vi "FPGA VeriStand Native DMA Interface.vi"() -> ()   [LabVIEW 2017]
uses:
  <vilib>/Platform/TimedLoop/XDataNode/timing_clust.ctl
  <vilib>/Platform/TimedLoop/XDataNode/nitl_modes.ctl
  <vilib>/Platform/TimedLoop/XDataNode/wakeup.ctl
  <vilib>/rvi/Emulation/niFpgaSctlEmulationGetInTimedLoop.vi
  <vilib>/rvi/Emulation/niFpgaEmulationReportErrorSimple.vi
  <vilib>/rvi/Emulation/niFpgaGetClockAttributes.vi
  <vilib>/rvi/Emulation/niFpgaCriticalErrorInLSC.vi
  <vilib>/rvi/eio/common/nirviEmuTemplateMethod_errors.vi
  <vilib>/rvi/Emulation/niFpgaProcessEmulError.vi
  <vilib>/Platform/TimedLoop/XDataNode/XDataNode.xnode
  <vilib>/eio/EIONode/EIONode.xnode
  <vilib>/eio/EIOMethodNode/EIOMethodNode.xnode
  <vilib>/Platform/TimedLoop/XDataNode/XDNodeRunTimeDep.lvlib
  <vilib>/NI Veristand/FPGA/NI_VS FPGA Support.lvlib
panel:
  in  "Generate IRQ":bool
  in  "Clock Pulse":bool
  in  "Clock Ticked":bool
  in  "Use External Timing":bool
  in  "Write to  RTSI":bool
  in  "Loop Rate (usec)":u32
  in  "Start":bool
  in  "_PWM In 1 timeout":u32=40000
  out "_PWM In 1 High Time":u32
  out "_PWM In 1 Low Time":u32
  in  "_PWM In 0 timeout":u32=40000
  out "_PWM In 0 High Time":u32
  out "_PWM In 0 Low Time":u32
  in  "_Low Pulse 1":u32
  in  "_High Pulse 1":u32
  in  "_Low Pulse 0":u32
  in  "_High Pulse 0":u32
  # "PWM"
  # "Configuration"
  # "Internal Controls"
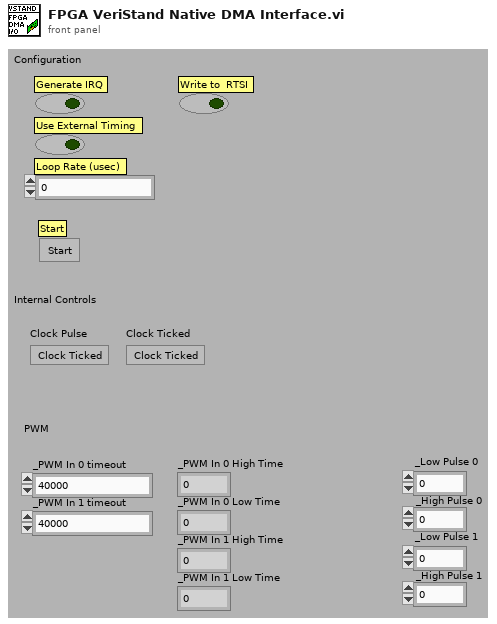
[diagram p1: front panel]
types:
  T1 = typedef "XDNodeRunTimeDep.lvlib/timing_clust.ctl" = cluster{"Expected End [f-1]":u64, "Actual End [f-1]":u64, "Finished Late? [f-1]":bool, "Expected End [i-1]":u64, "Actual End [i-1]":u64, "Finished Late? [i-1]":bool, "Expected Start [i]":u64, "Actual Start [i]":u64, "Expected Start [f]":u64, "Actual Start [f]":u64, "Source Name":string, "Structure Name":string, "Period":i64, "Deadline":i64, "Offset":i64, "Start":i64, "Priority":i32, "Timeout":i32, "Mode":T2, "Wakeup Reason":T3, "Error":errorcluster, "Source Type":string, "Secondary Source Type":string, "Global End Time":u64, "Global Start Time":u64, "Frame Duration":u64, "Iteration Duration":u64, "Assigned CPU":i32, "I/O Scan Engine Mode":u32}
  T2 = typedef "XDNodeRunTimeDep.lvlib/nitl_modes.ctl" = enum32{"No Change", "Process missed periods, maintain original phase", "Discard missed periods, maintain original phase", "Process missed periods, ignore original phase", "Discard missed periods, ignore original phase"}
  T3 = typedef "XDNodeRunTimeDep.lvlib/wakeup.ctl" = enum32{"Normal", "Aborted", "Asynchronous wakeup", "Timing source error", "Timed loop error", "Timeout"}
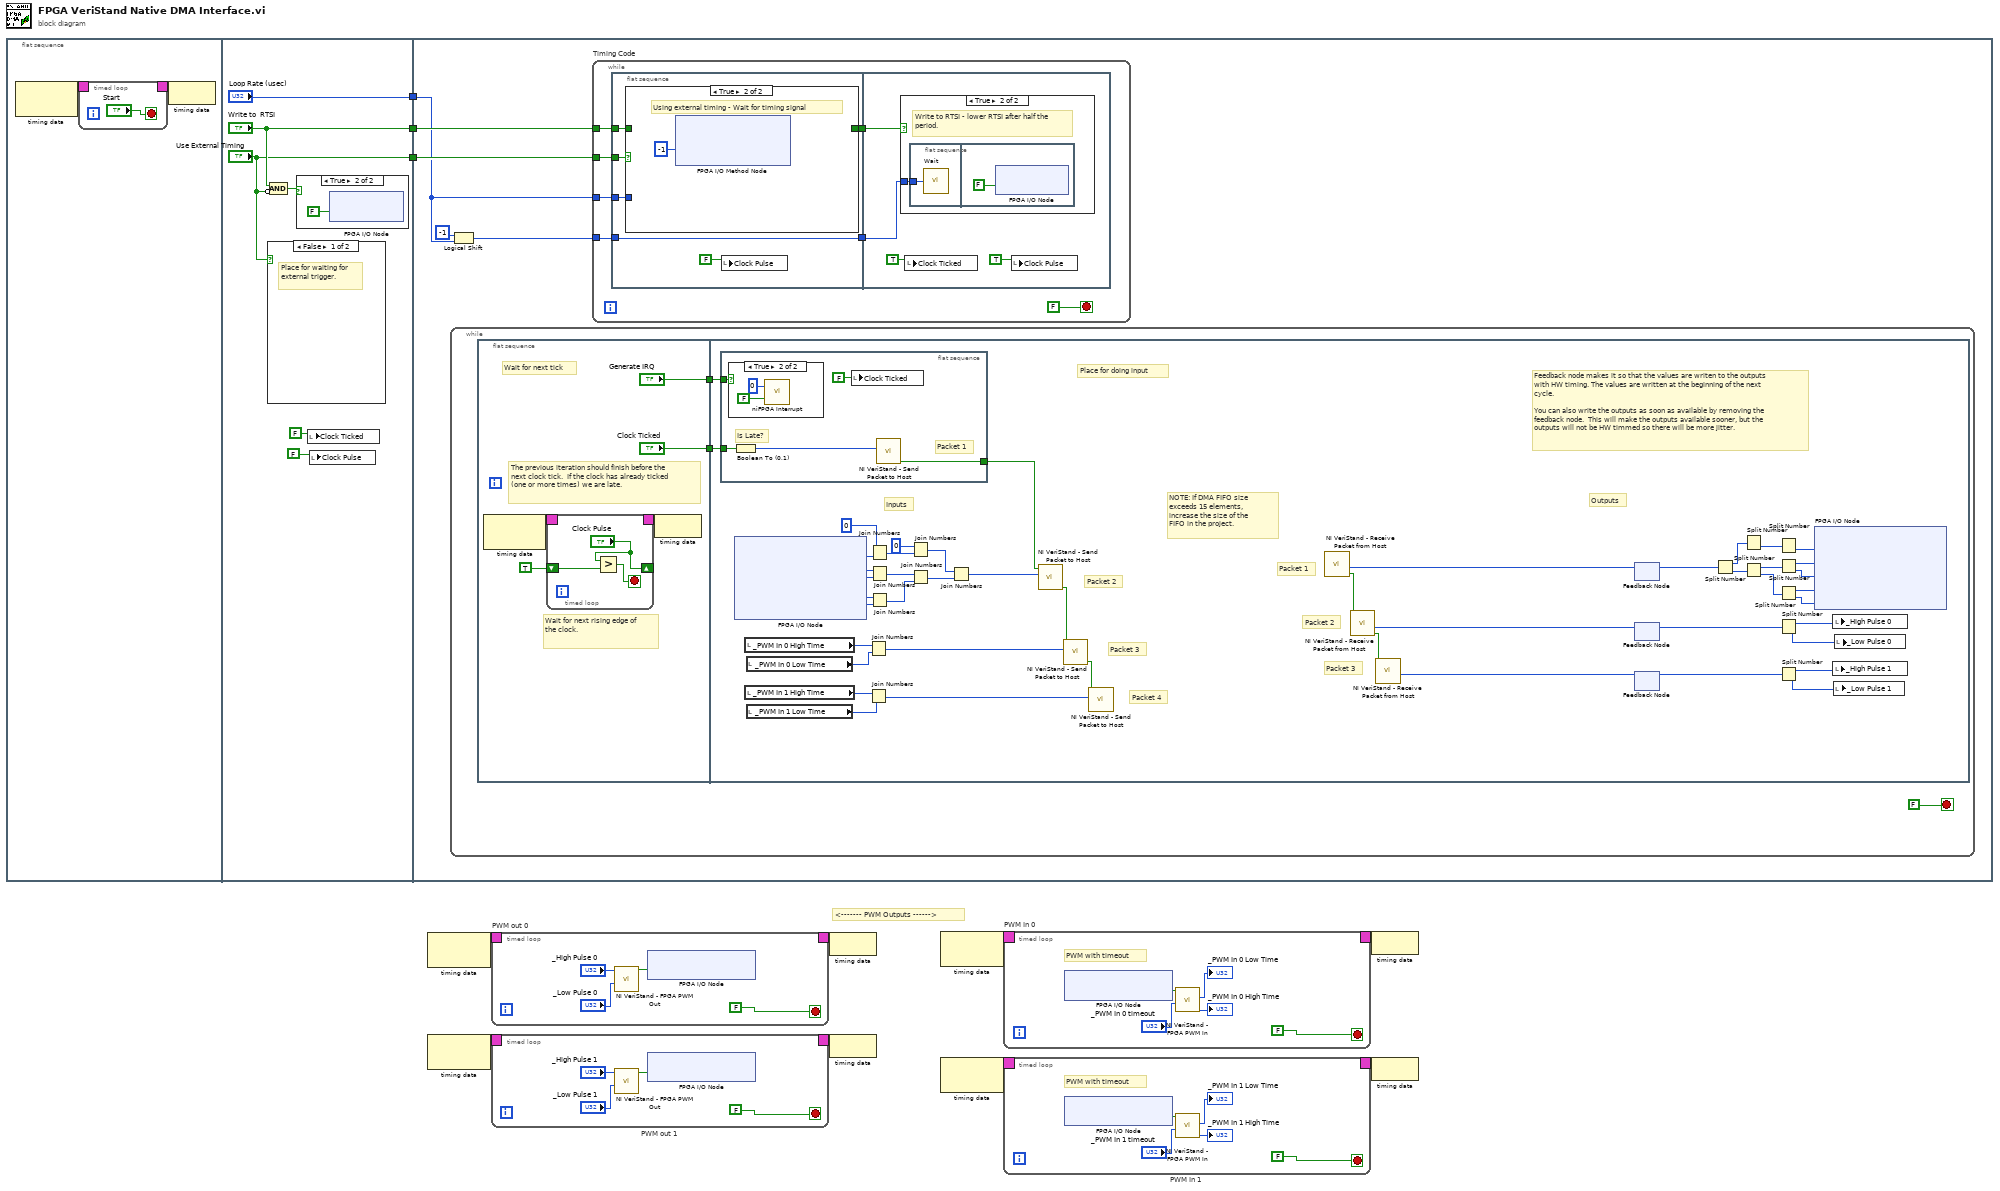
[diagram p0: block diagram]
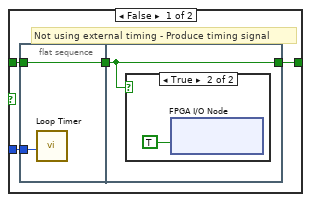
[diagram p4: hidden frame]
diagram:
  # "<------- PWM Outputs ------>"
  n1 = flat-sequence {
    tunnel: ["Use External Timing"] -> w3
    tunnel: ["Write to  RTSI"] -> w2
    tunnel: ["Loop Rate (usec)"] -> w1
    tunnel: w3 -> [w28]
    tunnel: w2 -> [w27]
    tunnel: w1 -> [w26]
    frame #0 {
      n2 = node-c288() -> (w13:T1)  [unwired: 1 out]
      n3 = timed-loop {
        timing: w13 -> [_]
        timing-out: [_] -> w12
        stop <- "Start" stop-if-true
      }
      n4 = node-c288(w12) -> ()
    }
    frame #1 {
      n5 = case shown="False" "Use External Timing" {
        frame False {
          # "Place for waiting for external trigger."
        }
        frame True {
          # "Do not wait on trigger when externally timed."
        }
      }
      n6 = Compound Arithmetic op=AND("Write to  RTSI", invert "Use External Timing") -> (w23:bool)
      n7 = case shown="True" w23 {
        frame False {
        }
        frame True {
          n8 = xnode "FPGA I/O Node"("PXI_Trig0"=FALSE ("TRIG0")) -> ()  [unwired: 1 in, 1 out]
        }
      }
      n9 = local write "Clock Ticked"(FALSE ("Clock Ticked")) -> ()
      n10 = local write "Clock Pulse"(FALSE ("Clock Ticked")) -> ()
    }
    frame #2 {
      n11 = Logical Shift(y=i8 -1, x=w26) -> (x << y=w29:u32)
      n12 = while {
        stop <- FALSE stop-if-true
        n13 = flat-sequence {
          tunnel: ["Generate IRQ"] -> w61
          tunnel: ["Clock Ticked"] -> w60
          tunnel: w61 -> [w120]
          tunnel: w60 -> [w119]
          frame #0 {
            # "The previous iteration should finish before the next clock tick.  If the clock has already ticked (one or more times) we are late."
            # "Wait for next rising edge of the clock."
            # "Wait for next tick"
            n14 = node-c288() -> (w66:T1)  [unwired: 1 out]
            n15 = timed-loop {
              timing: w66 -> [_]
              timing-out: [_] -> w65
              shift-right: ["Clock Pulse"] -> _
              shift-left: TRUE ("Clock Ticked") -> [w70]
              stop <- w69 stop-if-true
              n16 = Greater?(x="Clock Pulse", y=w70) -> (0:w69:bool)
            }
            n17 = node-c288(w65) -> ()
          }
          frame #1 {
            # "Inputs"
            # "Outputs"
            # "Packet 4"
            # "Packet 3"
            # "Packet 2"
            # "Packet 3"
            # "Packet 2"
            # "Packet 1"
            # "NOTE: If DMA FIFO size exceeds 15 elements, increase the size of the FIFO in the project."
            # "Feedback node makes it so that the values are writen to the outputs with HW timing. The values are written at the beginning of the next cycle.  \n\nYou can also write the outputs as soon as available by removing the feedback node.  This will make the outputs available sooner, but the outputs will not be HW timmed so there will be more jitter."
            # "Place for doing input"
            n18 = flat-sequence {
              tunnel: w120 -> [w125]
              tunnel: [w123] -> w75
              tunnel: w119 -> [w121]
              frame #0 {
                # "Packet 1"
                # "Is Late?"
                n19 = case shown="True" w125 {
                  frame False {
                  }
                  frame True {
                    n20 = call <vilib>:"niFPGA Interrupt.vi"("Wait Until Cleared (F)"=FALSE ("Wait Until Cleared"), "IRQ Number (0)"=u8 0 ("IRQ Number")) -> ()  [unwired: 1 in]
                  }
                }
                n21 = Boolean To (0,1)(Boolean=w121) -> (0, 1=w124:i16)
                n22 = local write "Clock Ticked"(FALSE ("Clock Ticked")) -> ()
                n23 = call <vilib>:"NI VeriStand - Send Packet to Host.vi"("Element"=w124) -> ("Next"=w123:bool)  [unwired: 1 in, 9 out]
              }
            }
            n24 = xnode "FPGA I/O Node"() -> ("Connector1/DIOPORT3"=w118:u8, "Connector1/DIOPORT3"=w117:u8, "Connector1/DIOPORT2"=w116:u8, "Connector1/DIOPORT1"=w115:u8, "Connector1/DIOPORT0"=w114:u8)  [unwired: 5 in, 5 out]
            n25 = local read "_PWM In 0 High Time"() -> (w108:u32)
            n26 = local read "_PWM In 1 High Time"() -> (w106:u32)
            n27 = local read "_PWM In 0 Low Time"() -> (w107:u32)
            n28 = local read "_PWM In 1 Low Time"() -> (w105:u32)
            n29 = Join Numbers(hi=w108, lo=w107) -> ((hi.lo)=w87:u64)
            n30 = Join Numbers(hi=w106, lo=w105) -> ((hi.lo)=w86:u64)
            n31 = Join Numbers(hi=u8 0, lo=w118) -> ((hi.lo)=w113:u16)
            n32 = Join Numbers(hi=w117, lo=w116) -> ((hi.lo)=w112:u16)
            n33 = Join Numbers(hi=w115, lo=w114) -> ((hi.lo)=w111:u16)
            n34 = Join Numbers(hi=u16 0, lo=w113) -> ((hi.lo)=w110:u32)
            n35 = Join Numbers(hi=w112, lo=w111) -> ((hi.lo)=w109:u32)
            n36 = Join Numbers(hi=w110, lo=w109) -> ((hi.lo)=w88:u64)
            n37 = call <vilib>:"NI VeriStand - Send Packet to Host.vi"("Element"=w88, "Prev"=w75) -> ("Next"=w77:bool)  [unwired: 1 in, 8 out]
            n38 = call <vilib>:"NI VeriStand - Send Packet to Host.vi"("Element"=w87, "Prev"=w77) -> ("Next"=w76:bool)  [unwired: 1 in, 8 out]
            n39 = call <vilib>:"NI VeriStand - Send Packet to Host.vi"("Element"=w86, "Prev"=w76) -> ()  [unwired: 1 in, 9 out]
            n40 = call <vilib>:"NI VeriStand - Receive Packet from Host.vi"() -> ("Next"=w79:bool, "Element"=w85:u64)  [unwired: 2 in, 8 out]
            n41 = call <vilib>:"NI VeriStand - Receive Packet from Host.vi"("Prev"=w79) -> ("Next"=w78:bool, "Element"=w84:u64)  [unwired: 1 in, 8 out]
            n42 = call <vilib>:"NI VeriStand - Receive Packet from Host.vi"("Prev"=w78) -> ("Element"=w83:u64)  [unwired: 1 in, 9 out]
            n43 = feedback-in #1(w85) -> ()
            n44 = feedback #1() -> (w82:u64)  [unwired: 1 out]
            n45 = feedback-in #2(w84) -> ()
            n46 = feedback #2() -> (w81:u64)  [unwired: 1 out]
            n47 = feedback-in #3(w83) -> ()
            n48 = feedback #3() -> (w80:u64)  [unwired: 1 out]
            n49 = Split Number(x=w82) -> (hi(x)=w99:u32, lo(x)=w98:u32)
            n50 = Split Number(x=w99) -> (lo(x)=w100:u16)  [unwired: 1 out]
            n51 = Split Number(x=w98) -> (hi(x)=w102:u16, lo(x)=w101:u16)
            n52 = Split Number(x=w100) -> (lo(x)=w89:u8)  [unwired: 1 out]
            n53 = Split Number(x=w102) -> (hi(x)=w90:u8, lo(x)=w91:u8)
            n54 = Split Number(x=w101) -> (hi(x)=w92:u8, lo(x)=w93:u8)
            n55 = Split Number(x=w81) -> (hi(x)=w97:u32, lo(x)=w96:u32)
            n56 = Split Number(x=w80) -> (hi(x)=w95:u32, lo(x)=w94:u32)
            n57 = xnode "FPGA I/O Node"("Connector0/DIOPORT0"=w89, "Connector0/DIOPORT1"=w90, "Connector0/DIOPORT0"=w91, "Connector0/DIOPORT1"=w92, "Connector0/DIOPORT0"=w93) -> ()  [unwired: 5 in, 5 out]
            n58 = local write "_High Pulse 0"(w97) -> ()
            n59 = local write "_High Pulse 1"(w95) -> ()
            n60 = local write "_Low Pulse 1"(w94) -> ()
            n61 = local write "_Low Pulse 0"(w96) -> ()
          }
        }
      }
      n62 = while "Timing Code" {
        tunnel: w29 -> [w37]
        tunnel: w26 -> [w36]
        tunnel: w28 -> [w35]
        tunnel: w27 -> [w34]
        stop <- FALSE stop-if-true
        n63 = flat-sequence {
          tunnel: w37 -> [w40]
          tunnel: w36 -> [w43]
          tunnel: w35 -> [w42]
          tunnel: w34 -> [w41]
          tunnel: [w40] -> w32
          tunnel: [w38] -> w31
          tunnel: w32 -> [w56]
          tunnel: w31 -> [w53]
          frame #0 {
            n64 = case shown="True" w42 {
              tunnel: w43 -> [w47 _]
              tunnel: w41 -> [w45 _]
              tunnel: [w44 _] -> w38
              frame False {
                # "Not using external timing - Produce timing signal"
                n65 = flat-sequence {
                  tunnel: [w48] -> w46
                  tunnel: w47 -> [w49]
                  tunnel: w45 -> [w48]
                  tunnel: w46 -> [w50]
                  tunnel: [w50] -> w44
                  frame #0 {
                    n66 = call "Loop Timer"("Count(uSec)"=w49) -> ()  [unwired: 1 out]
                  }
                  frame #1 {
                    n67 = case shown="True" w50 {
                      frame False {
                      }
                      frame True {
                        n68 = xnode "FPGA I/O Node"("PXI_Trig0"=TRUE ("TRIG0")) -> ()  [unwired: 1 in, 1 out]
                      }
                    }
                  }
                }
              }
              frame True {
                # "Using external timing - Wait for timing signal"
                n69 = xnode "FPGA I/O Method Node"("Timeout"=-1) -> ()  [unwired: 1 in, 2 out]
              }
            }
            n70 = local write "Clock Pulse"(FALSE ("Clock Ticked")) -> ()
          }
          frame #1 {
            n71 = case shown="True" w53 {
              tunnel: w56 -> [_ w57]
              frame False {
              }
              frame True {
                # "Write to RTSI - lower RTSI after half the period."
                n72 = flat-sequence {
                  tunnel: w57 -> [w58]
                  frame #0 {
                    n73 = call "Wait"("Count(uSec)"=w58) -> ()  [unwired: 1 out]
                  }
                  frame #1 {
                    n74 = xnode "FPGA I/O Node"("PXI_Trig0"=FALSE ("TRIG0")) -> ()  [unwired: 1 in, 1 out]
                  }
                }
              }
            }
            n75 = local write "Clock Ticked"(TRUE ("Clock Ticked")) -> ()
            n76 = local write "Clock Pulse"(TRUE ("Clock Ticked")) -> ()
          }
        }
      }
    }
  }
  n77 = node-c288() -> (w11:T1)  [unwired: 1 out]
  n78 = node-c288() -> (w9:T1)  [unwired: 1 out]
  n79 = timed-loop "PWM out 0" {
    timing: w11 -> [_]
    timing-out: [_] -> w10
    stop <- FALSE stop-if-true
    n80 = call <vilib>:"NI VeriStand - FPGA PWM Out.vi"("_Low Time"="_Low Pulse 0", "_High Time"="_High Pulse 0") -> ("Output"=w130:bool)  [unwired: 1 in, 8 out]
    n81 = xnode "FPGA I/O Node"("Connector0/DIO4"=w130) -> ()  [unwired: 1 in, 1 out]
  }
  n82 = timed-loop "PWM out 1" {
    timing: w9 -> [_]
    timing-out: [_] -> w8
    stop <- FALSE stop-if-true
    n83 = call <vilib>:"NI VeriStand - FPGA PWM Out.vi"("_Low Time"="_Low Pulse 1", "_High Time"="_High Pulse 1") -> ("Output"=w134:bool)  [unwired: 1 in, 8 out]
    n84 = xnode "FPGA I/O Node"("Connector0/DIO5"=w134) -> ()  [unwired: 1 in, 1 out]
  }
  n85 = node-c288(w10) -> ()
  n86 = node-c288(w8) -> ()
  n87 = node-c288() -> (w7:T1)  [unwired: 1 out]
  n88 = node-c288() -> (w5:T1)  [unwired: 1 out]
  n89 = timed-loop "PWM In 0" {
    timing: w7 -> [_]
    timing-out: [_] -> w6
    stop <- FALSE stop-if-true
    # "PWM with timeout"
    n90 = xnode "FPGA I/O Node"() -> ("Connector0/DIO0"=w143:bool)  [unwired: 1 in, 1 out]
    n91 = call <vilib>:"NI VeriStand - FPGA PWM In.vi"("Time Out"="_PWM In 0 timeout", "Value"=w143) -> ("High time"=→"_PWM In 0 High Time":u32, "Low Time"=→"_PWM In 0 Low Time":u32)  [unwired: 8 out]
  }
  n92 = timed-loop "PWM In 1" {
    timing: w5 -> [_]
    timing-out: [_] -> w4
    stop <- FALSE stop-if-true
    # "PWM with timeout"
    n93 = xnode "FPGA I/O Node"() -> ("Connector0/DIO1"=w150:bool)  [unwired: 1 in, 1 out]
    n94 = call <vilib>:"NI VeriStand - FPGA PWM In.vi"("Time Out"="_PWM In 1 timeout", "Value"=w150) -> ("High time"=→"_PWM In 1 High Time":u32, "Low Time"=→"_PWM In 1 Low Time":u32)  [unwired: 8 out]
  }
  n95 = node-c288(w6) -> ()
  n96 = node-c288(w4) -> ()
